vi "Message.vi"(8 "error in (no error)":errorcluster, 9 "Enable":bool=TRUE, 10 "Message":string) -> (0 "error out":errorcluster, 2 "OK":bool)   [LabVIEW 2014]
doc: "Displays a standard dialog box that contains an alert or a message for users.\n--------------------\n\nThis Express VI is configured as follows:\n\nMessage:"
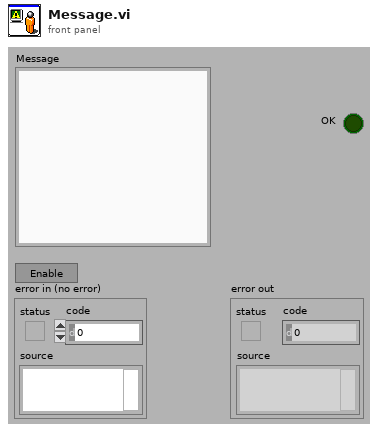
[diagram p1: front panel]
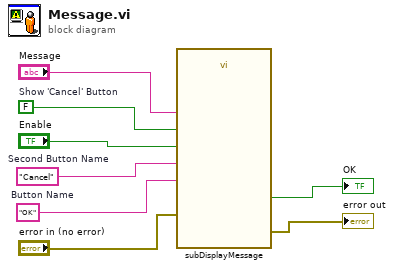
[diagram p0: block diagram]
diagram:
  w3 = "OK"  # Button Name
  w4 = "Cancel"  # Second Button Name
  w6 = FALSE  # Show 'Cancel' Button
  n1 = call <vilib>:"subDisplayMessage.vi"("Second Button Name"=w4, "Button Name"=w3, "error in (no error)"="error in (no error)", "Enable Message"="Enable", "Show 'Cancel' Button"=w6, "Message to Display"="Message") -> ("error out"=→"error out":errorcluster, "OK?"=→"OK":bool)  [unwired: 4 in]
